vi "Stop Motion.vi"(8 "error in (no error)":errorcluster, 11 "2-Axis Stage in":refnum<class "XY Stage Process.lvclass">) -> (0 "error out":errorcluster, 3 "2-Axis Stage out":refnum<class "XY Stage Process.lvclass">)   [LabVIEW 2022 SP3, in "XY Stage Process.lvlib" / "XY Stage Process.lvclass"]
uses:
  XY Stage Process.lvclass
  XY Stage Process.lvclass/XY Stage Process.ctl
  Process Framework/Process State Data/Process State Data.lvclass/Process State Data.ctl
  Process Framework/Process State Data/Accessor/Write Abort.vi
  Process Framework/Process State Data/Process State Data.lvclass
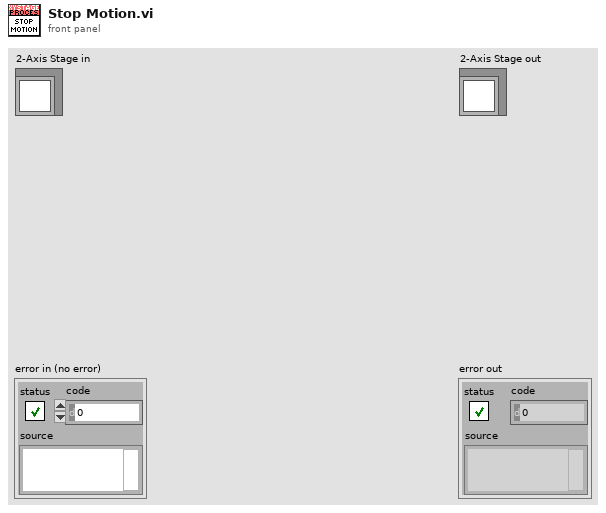
[diagram p1: front panel]
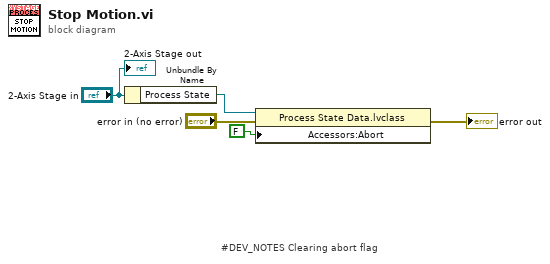
[diagram p0: block diagram]
diagram:
  # "#DEV_NOTES Clearing abort flag"
  n1 = Unbundle By Name("2-Axis Stage in") -> ("Process State"=w4:refnum<data-value>)
  n2 = property class="Process State Data.lvclass"(reference=w4, error in="error in (no error)", "Accessors:Abort"=FALSE ("Abort")) -> (error out=→"error out":errorcluster)  [unwired: 1 out]
  "2-Axis Stage out" <- "2-Axis Stage in"
